vi "Compute.vi"(8 "error in (no error)":errorcluster, 9 "Data Channels":T3, 10 "x-var":T2(array[cluster]), 11 "Norm in":refnum<class "Norm.lvclass">) -> (0 "error out":errorcluster, 1 "Add'l Data Channels":T3, 3 "Norm out":refnum<class "Norm.lvclass">)   [LabVIEW 2015, in "Norm.lvclass"]
doc: "Given a data channel and an x-coordinate, compute and return one or more new data channels."
uses:
  Norm.lvclass
  Instruments/Utility Classes/Readable/Data Channels.ctl
  Instruments/Utility Classes/Readable/Data Channel.ctl
  Instruments/Utility Classes/Readable/Data Point.ctl
  Instruments/Utility Classes/Readable/Time.ctl
  Instruments/Utility Classes/Readable/X.ctl
  Instruments/Utility Classes/Readable/Readable.lvclass
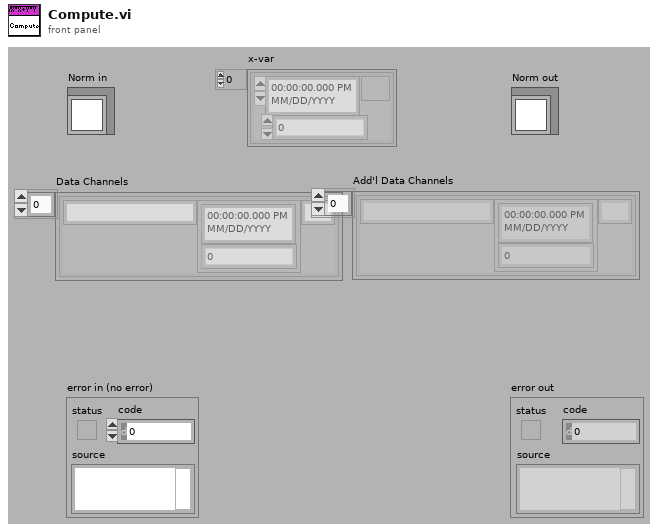
[diagram p1: front panel]
types:
  T1 = typedef "Readable.lvclass/X.ctl" = dbl
  T2 = cluster{"seconds since 1Jan1904":timestamp, "X-Var":T1}[]
  T3 = typedef "Readable.lvclass/Data Channels.ctl" = T4[]
  T4 = typedef "Readable.lvclass/Data Channel.ctl" = cluster{"Name":string, "Data Point":T5, "Unit":string}
  T5 = typedef "Readable.lvclass/Data Point.ctl" = cluster{"t":T6, "x":T1}
  T6 = typedef "Readable.lvclass/Time.ctl" = timestamp
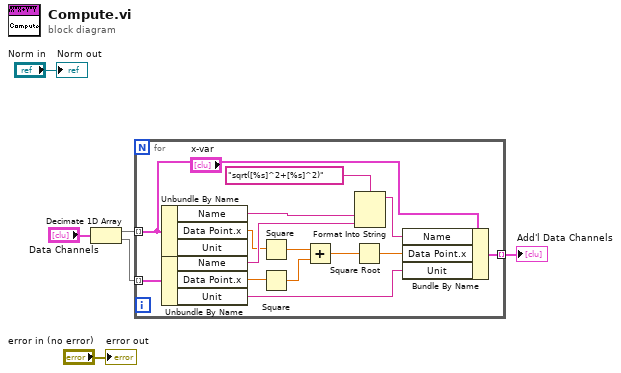
[diagram p0: block diagram]
diagram:
  n1 = Decimate 1D Array("Data Channels") -> (w6:T4[], w5:T4[])
  n2 = for {
    tunnel: w6 -> [w16] mode=indexing
    tunnel: w5 -> [w20] mode=indexing
    tunnel: [w12] -> w3 mode=indexing
    n3 = Unbundle By Name(w16) -> ("Name"=w18:string, "Data Point.x"=w8:T1)  [unwired: 1 out]
    n4 = Unbundle By Name(w20) -> ("Name"=w17:string, "Data Point.x"=w9:T1, "Unit"=w15:string)
    n5 = Square(x=w8) -> (x^2=w11:T1)
    n6 = Square(x=w9) -> (x^2=w10:T1)
    n7 = Add(x=w11, y=w10) -> (x+y=w13:T1)
    n8 = Square Root(x=w13) -> (sqrt(x)=w7:T1)
    n9 = Format Into String(format string="sqrt([%s]^2+[%s]^2)", w18, w17) -> (resulting string=w14:string)  [unwired: 2 in, 1 out]
    n10 = Bundle By Name(cluster=w16, "Name"=w14, "Data Point.x"=w7, "Unit"=w15) -> (w12:T4)
  }
  "Add'l Data Channels" <- w3
  "error out" <- "error in (no error)"
  "Norm out" <- "Norm in"
